vi "write.vi"   [LabVIEW 2012]
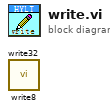
[diagram p0: block diagram]
diagram:
  n1 = call "write8.vi"() -> ()  [unwired: 10 in, 2 out]
  n2 = call "write32.vi"() -> ()  [unwired: 10 in, 2 out]
